vi "Thorlabs Translation Stage Module.vi"(7 "Action":T1, 8 "error in (no error)":errorcluster, 9 "Cluster In":T3, 10 "Set/Get":T2, 11 ".NET Refnum in":refnum<k24>) -> (0 "error out":errorcluster, 2 "Cluster out":T3, 3 ".NET Refnum out":refnum<k24>)   [LabVIEW 2018]
uses:
  C:/Project/SSOCT/Labview Software/Thorlabs.MotionControl.Controls.dll
  Thorlabs.MotionControl.Controls.dll
  Hardware Mfg/Thorlabs Translation Stages/Controls/Translation Stage Cluster.ctl
  Controls/Translation Stage Types.ctl
  Controls/Set Get Controls.ctl
  Hardware Mfg/Thorlabs Translation Stages/Controls/Motion Translation Module Control2.ctl
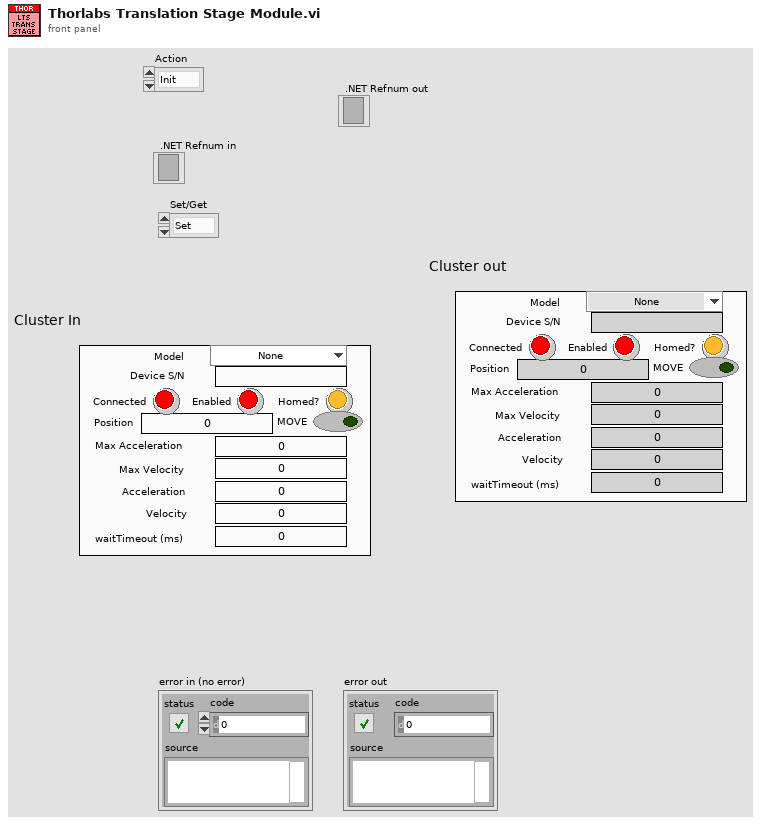
[diagram p1: front panel]
types:
  T1 = typedef "Motion Translation Module Control2.ctl" = enum16{"Init", "Home", "Status", "Velocity/Accel", "Position", "Jog", "Stop", "Uninit", "Enable", "Disable"}
  T2 = typedef "Set Get Controls.ctl" = enum16{"Set", "Get"}
  T3 = typedef "Translation Stage Cluster.ctl" = cluster{"Position":dbl, "Is.Enabled?":bool, "Is.Connected?":bool, "Device SN":string, "AccelerationMaximum":dbl, "VelocityMaximum":dbl, "Acceleration":dbl, "Velocity":dbl, "waitTimeout (ms)":i32, "Model":T4, "Is.Homed?":bool, "MOVE":bool}
  T4 = typedef "Translation Stage Types.ctl" = enum16{"None", "Thorlabs LTS", "Thorlabs MLJ"}
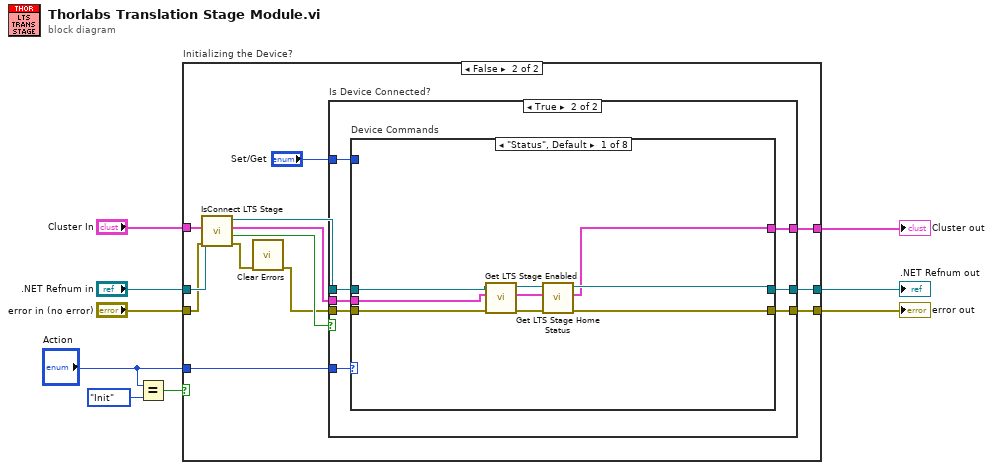
[diagram p0: block diagram]
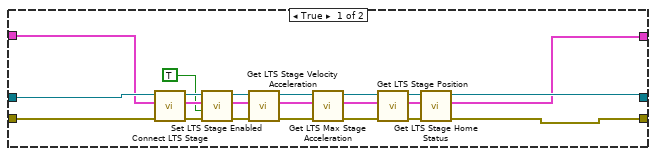
[diagram p2: hidden frame]
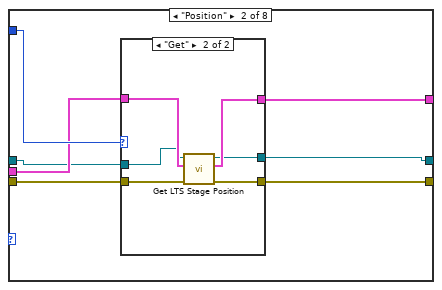
[diagram p4: hidden frame]
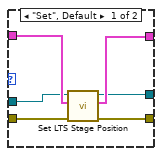
[diagram p5: hidden frame]
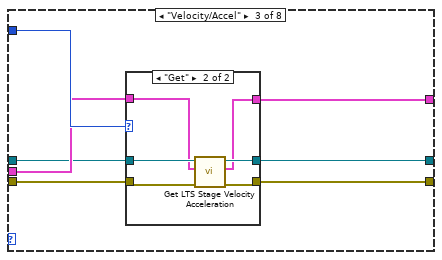
[diagram p6: hidden frame]
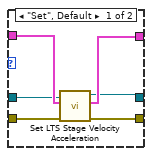
[diagram p7: hidden frame]
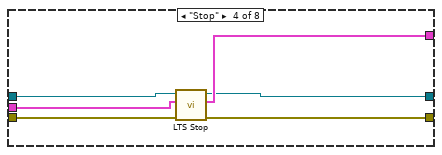
[diagram p8: hidden frame]
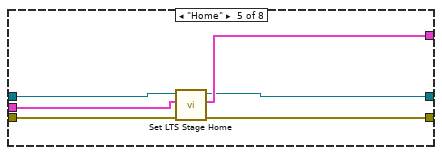
[diagram p9: hidden frame]
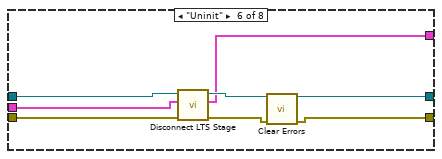
[diagram p10: hidden frame]
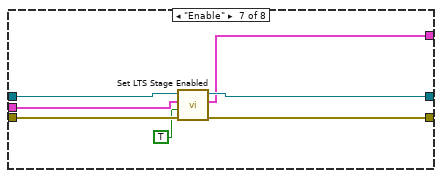
[diagram p11: hidden frame]
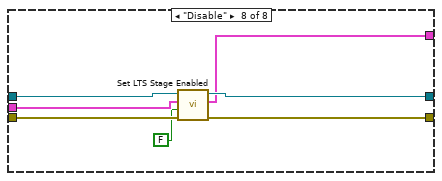
[diagram p12: hidden frame]
diagram:
  n1 = Equal?(x="Action", y=Motion_Translation_Module_Control2."Init" ("Action")) -> (x = y?=w3:bool)
  n2 = case "Initializing the Device?" shown="False" w3 {
    tunnel: ".NET Refnum in" -> [w31 w39]
    tunnel: [w19 w44] -> w8
    tunnel: [w18 w43] -> w7
    tunnel: [w11 w42] -> w6
    tunnel: "error in (no error)" -> [w10 w33]
    tunnel: "Cluster In" -> [w30 w36]
    tunnel: "Action" -> [_ w41]
    frame True {
      n3 = call "Connect LTS Stage.vi"("error in (no error)"=w10, "Cluster in"=w30, "LTS Reference In"=w31) -> ("error out"=w29:errorcluster, "Cluster out"=w27:T3, "LTS Reference Out"=w28:refnum<k24>)  [unwired: 5 in, 1 out]
      n4 = call "Set LTS Stage Enabled.vi"("error in (no error)"=w29, "Enable?"=TRUE, "Cluster in"=w27, "LTS Reference In"=w28) -> ("error out"=w26:errorcluster, "Cluster out"=w25:T3, "LTS Reference Out"=w24:refnum<k24>)  [unwired: 5 in]
      n5 = call "Get LTS Stage Velocity Acceleration.vi"("error in (no error)"=w26, "Cluster in"=w25, "LTS Reference In"=w24) -> ("error out"=w23:errorcluster, "Cluster out"=w15:T3, "LTS Reference Out"=w14:refnum<k24>)  [unwired: 5 in, 1 out]
      n6 = call "Get LTS Max Stage Acceleration.vi"("error in (no error)"=w23, "Cluster in"=w15, "LTS Reference In"=w14) -> ("error out"=w16:errorcluster, "Cluster out"=w12:T3, "LTS Reference Out"=w13:refnum<k24>)  [unwired: 4 in, 2 out]
      n7 = call "Get LTS Stage Position.vi"("error in (no error)"=w16, "Cluster in"=w12, "LTS Reference In"=w13) -> ("error out"=w22:errorcluster, "Cluster out"=w21:T3, "LTS Reference Out"=w20:refnum<k24>)  [unwired: 5 in, 1 out]
      n8 = call "Get LTS Stage Home Status.vi"("error in (no error)"=w22, "Cluster in"=w21, "LTS Reference In"=w20) -> ("error out"=w11:errorcluster, "Cluster out"=w18:T3, "LTS Reference Out"=w19:refnum<k24>)  [unwired: 6 in]
    }
    frame False {
      n9 = call "IsConnect LTS Stage.vi"("error in (no error)"=w33, "Cluster in"=w36, "LTS Reference In"=w39) -> ("error out"=w34:errorcluster, "IsConnected"=w37:bool, "Cluster out"=w35:T3, "LTS Reference Out"=w38:refnum<k24>)  [unwired: 5 in]
      n10 = call <vilib>:"Clear Errors.vi"("error in (no error)"=w34) -> ("error out"=w32:errorcluster)  [unwired: 5 in, 1 out]
      n11 = case "Is Device Connected?" shown="True" w37 {
        tunnel: w38 -> [w45 w55]
        tunnel: [w45 w54] -> w44
        tunnel: [w47 w53] -> w43
        tunnel: [w46 w52] -> w42
        tunnel: w32 -> [w46 w51]
        tunnel: "Set/Get" -> [_ w50]
        tunnel: w41 -> [_ w49]
        tunnel: w35 -> [w47 w48]
        frame False {
        }
        frame True {
          n12 = case "Device Commands" shown="\"Status\", Default" w49 {
            tunnel: w50 -> [_ w71 w90 _ _ _ _ _]
            tunnel: w48 -> [w57 w68 w87 w106 w112 w119 w125 w132]
            tunnel: w51 -> [w58 w70 w89 w108 w114 w121 w128 w135]
            tunnel: [w61 w66 w85 w104 w110 w120 w126 w133] -> w54
            tunnel: [w62 w69 w88 w107 w113 w115 w127 w134] -> w52
            tunnel: [w59 w67 w86 w105 w111 w118 w124 w131] -> w53
            tunnel: w55 -> [w56 w65 w84 w103 w109 w117 w123 w130]
            frame "Status", Default {
              n13 = call "Get LTS Stage Enabled.vi"("error in (no error)"=w58, "Cluster in"=w57, "LTS Reference In"=w56) -> ("error out"=w64:errorcluster, "Cluster out"=w60:T3, "LTS Reference Out"=w63:refnum<k24>)  [unwired: 5 in, 1 out]
              n14 = call "Get LTS Stage Home Status.vi"("error in (no error)"=w64, "Cluster in"=w60, "LTS Reference In"=w63) -> ("error out"=w62:errorcluster, "Cluster out"=w59:T3, "LTS Reference Out"=w61:refnum<k24>)  [unwired: 6 in]
            }
            frame "Position" {
              n15 = case shown="\"Get\"" w71 {
                tunnel: w70 -> [w77 w83]
                tunnel: [w76 w82] -> w69
                tunnel: w68 -> [w75 w81]
                tunnel: [w74 w80] -> w67
                tunnel: w65 -> [w73 w79]
                tunnel: [w72 w78] -> w66
                frame "Set", Default {
                  n16 = call "Set LTS Stage Position.vi"("error in (no error)"=w77, "Cluster in"=w75, "LTS Reference In"=w73) -> ("error out"=w76:errorcluster, "Cluster out"=w74:T3, "LTS Reference Out"=w72:refnum<k24>)  [unwired: 6 in]
                }
                frame "Get" {
                  n17 = call "Get LTS Stage Position.vi"("error in (no error)"=w83, "Cluster in"=w81, "LTS Reference In"=w79) -> ("error out"=w82:errorcluster, "Cluster out"=w80:T3, "LTS Reference Out"=w78:refnum<k24>)  [unwired: 5 in, 1 out]
                }
              }
            }
            frame "Velocity/Accel" {
              n18 = case shown="\"Get\"" w90 {
                tunnel: w89 -> [w96 w102]
                tunnel: [w95 w101] -> w88
                tunnel: w87 -> [w93 w98]
                tunnel: [w94 w97] -> w86
                tunnel: w84 -> [w92 w99]
                tunnel: [w91 w100] -> w85
                frame "Set", Default {
                  n19 = call "Set LTS Stage Velocity Acceleration.vi"("error in (no error)"=w96, "Cluster in"=w93, "LTS Reference In"=w92) -> ("error out"=w95:errorcluster, "Cluster out"=w94:T3, "LTS Reference Out"=w91:refnum<k24>)  [unwired: 6 in]
                }
                frame "Get" {
                  n20 = call "Get LTS Stage Velocity Acceleration.vi"("error in (no error)"=w102, "Cluster in"=w98, "LTS Reference In"=w99) -> ("error out"=w101:errorcluster, "Cluster out"=w97:T3, "LTS Reference Out"=w100:refnum<k24>)  [unwired: 5 in, 1 out]
                }
              }
            }
            frame "Stop" {
              n21 = call "LTS Stop.vi"("error in (no error)"=w108, "Cluster in"=w106, "LTS Reference In"=w103) -> ("error out"=w107:errorcluster, "Cluster out"=w105:T3, "LTS Reference Out"=w104:refnum<k24>)  [unwired: 6 in]
            }
            frame "Home" {
              n22 = call "Set LTS Stage Home.vi"("error in (no error)"=w114, "Cluster in"=w112, "LTS Reference In"=w109) -> ("error out"=w113:errorcluster, "Cluster out"=w111:T3, "LTS Reference Out"=w110:refnum<k24>)  [unwired: 6 in]
            }
            frame "Uninit" {
              n23 = call "Disconnect LTS Stage.vi"("error in (no error)"=w121, "Cluster in"=w119, "LTS Reference In"=w117) -> ("error out"=w116:errorcluster, "Cluster out"=w118:T3, "LTS Reference Out"=w120:refnum<k24>)  [unwired: 6 in]
              n24 = call <vilib>:"Clear Errors.vi"("error in (no error)"=w116) -> ("error out"=w115:errorcluster)  [unwired: 5 in, 1 out]
            }
            frame "Enable" {
              n25 = call "Set LTS Stage Enabled.vi"("error in (no error)"=w128, "Enable?"=TRUE, "Cluster in"=w125, "LTS Reference In"=w123) -> ("error out"=w127:errorcluster, "Cluster out"=w124:T3, "LTS Reference Out"=w126:refnum<k24>)  [unwired: 5 in]
            }
            frame "Disable" {
              n26 = call "Set LTS Stage Enabled.vi"("error in (no error)"=w135, "Enable?"=FALSE, "Cluster in"=w132, "LTS Reference In"=w130) -> ("error out"=w134:errorcluster, "Cluster out"=w131:T3, "LTS Reference Out"=w133:refnum<k24>)  [unwired: 5 in]
            }
          }
        }
      }
    }
  }
  ".NET Refnum out" <- w8
  "Cluster out" <- w7
  "error out" <- w6
